vi "about get DD DF Version.vi"(8 "error in (no error)":errorcluster) -> (0 "error out":errorcluster, 2 "DF Version":T1 {"Build Date/Time" format="%<%X\n%x>T"}, 3 "DD Version":T1 {"Build Date/Time" format="%<%X\n%x>T"})   [LabVIEW 2011]
uses:
  Summitek EXT/Miscellaneous/OGAB Version.ctl
  Summitek EXT/OpenG EXT/file/file.llb/File Exists - Scalar__ogtk.vi
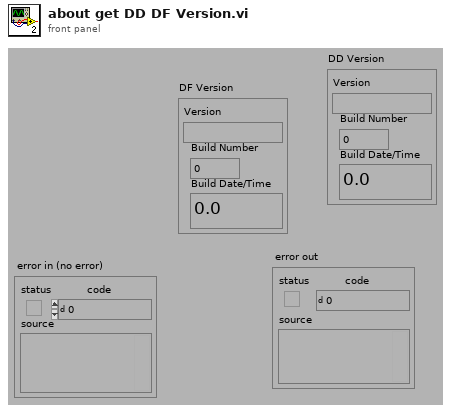
[diagram p1: front panel]
types:
  T1 = typedef "OGAB Version.ctl" = cluster{"Version":string, "Build Number":u32, "Build Date/Time":dbl}
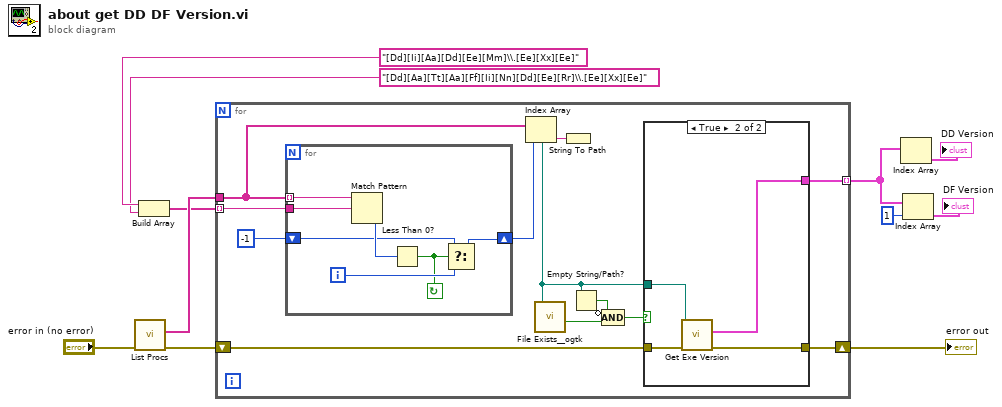
[diagram p0: block diagram]
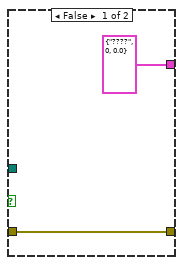
[diagram p2: hidden frame]
diagram:
  n1 = call "List Procs.vi"("error in (no error)"="error in (no error)") -> ("error out"=w6:errorcluster, "FullModuleNames"=w10:string[])  [unwired: 5 out]
  n2 = Build Array("[Dd][Ii][Aa][Dd][Ee][Mm]\\.[Ee][Xx][Ee]" ("regular expression"), "[Dd][Aa][Tt][Aa][Ff][Ii][Nn][Dd][Ee][Rr]\\.[Ee][Xx][Ee]" ("regular expression")) -> (w7:string[])
  n3 = for {
    tunnel: w10 -> [w22]
    tunnel: w7 -> [w20] mode=indexing
    shift-right: [w17] -> w5
    shift-left: w6 -> [w18]
    tunnel: [w16] -> w4 mode=indexing
    n4 = for {
      tunnel: w22 -> [w36] mode=indexing
      shift-right: [w33] -> w21
      shift-left: -1 -> [w34]
      tunnel: w20 -> [w30]
      i -> [w32]
      stop <- w31 continue-if-true
      n5 = Match Pattern(string=w36, regular expression=w30) -> (offset past match=w35:i32)  [unwired: 4 out]
      n6 = Less Than 0?(x=w35) -> (x < 0?=w31:bool)
      n7 = Select(t=w34, s=w31, f=w32) -> (s? t:f=w33:i32)
    }
    n8 = Index Array(array=w22, index=w21) -> (element=w19:string)
    n9 = String To Path(string=w19) -> (path=w15:path)
    n10 = call-poly "File Exists__ogtk.vi"("file path"=w15) -> ("exists"=w13:bool)  [unwired: 6 in, 1 out]
    n11 = Empty String/Path?(string/path=w15) -> (empty?=w14:bool)
    n12 = Compound Arithmetic op=AND(invert w14, w13) -> (w12:bool)
    n13 = case shown="True" w12 {
      tunnel: w18 -> [w25 w29]
      tunnel: w15 -> [_ w28]
      tunnel: [w25 w27] -> w17
      tunnel: [T1 {"Version"="????", "Build Number"=0, "Build Date/Time"=0.0} ("Version") w26] -> w16
      frame False {
      }
      frame True {
        n14 = call "Get Exe Version.vi"("error in (no error)"=w29, "EXE Path (\"\")"=w28) -> ("error out"=w27:errorcluster, "Version"=w26:T1)  [unwired: 8 out]
      }
    }
  }
  "error out" <- w5
  n15 = Index Array(array=w4) -> (element=→"DD Version":T1)  [unwired: 1 in]
  n16 = Index Array(array=w4, index=1) -> (element=→"DF Version":T1)
